vi "Y Axis Motor state control subVI.vi"(8 "error in (no error)":errorcluster, 11 "Y Axis Motor Target":T1) -> (0 "error out":errorcluster, 3 "Y Axis Motor Params":T2)   [LabVIEW 2017]
uses:
  X-Y Manipulator open loop/Control 1.ctl
  Motor Status Enum.ctl
panel:
  in  "Y Axis Motor Target":T1
  in  "stop":bool
  in  "stop 2":bool
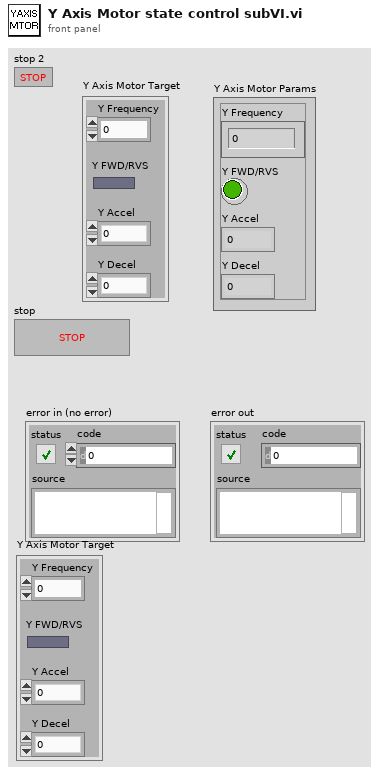
[diagram p1: front panel]
types:
  T1 = typedef "Control 1.ctl" = cluster{"Y Frequency":dbl, "Y FWD/RVS":bool, "Y Accel":dbl, "Y Decel":dbl}
  T2 = cluster{"Y Frequency":dbl, "Y FWD/RVS":bool, "Y Accel":dbl, "Y Decel":dbl}
  T3 = typedef "Motor Status Enum.ctl" = enum16{"Stop Motor", "Read Inputs", "Steady Speed", "Accelerate", "Decelerate"}
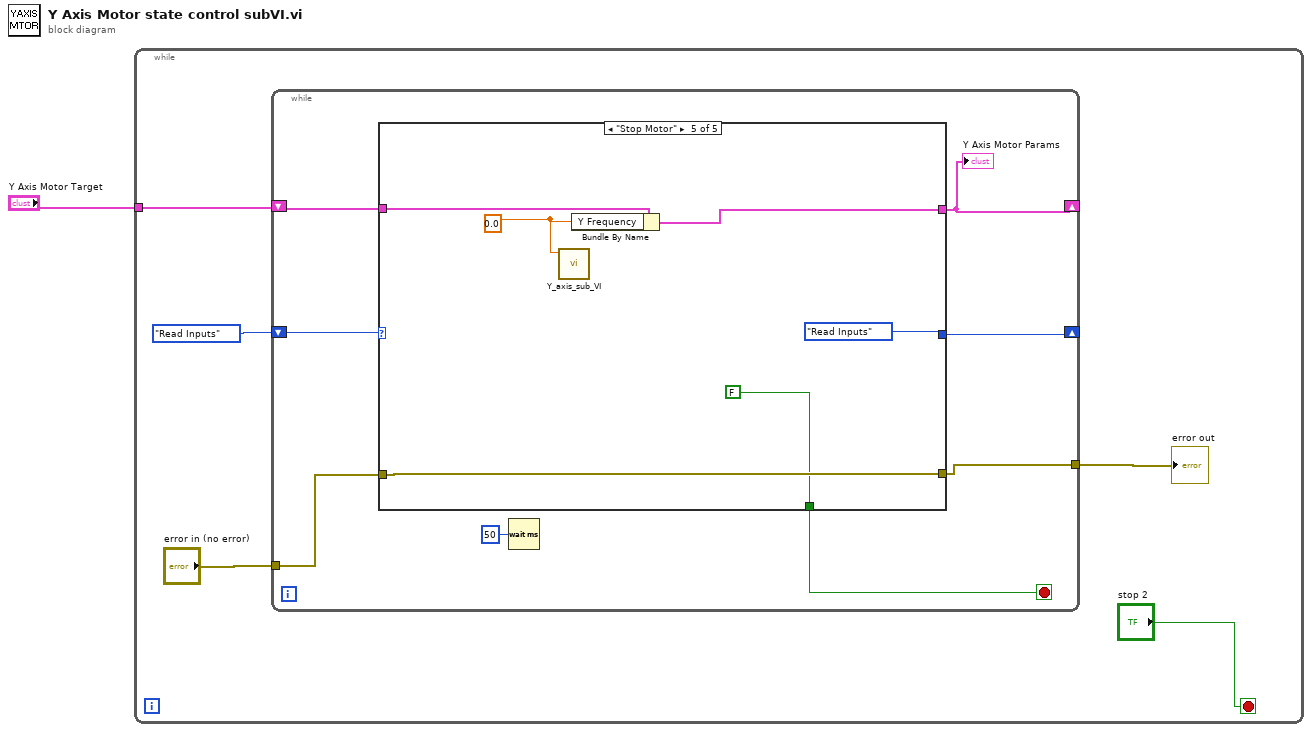
[diagram p0: block diagram]
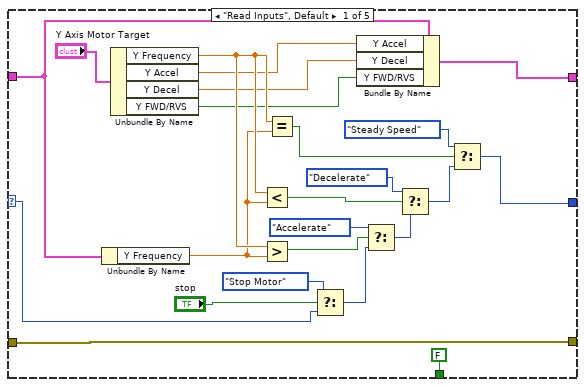
[diagram p2: hidden frame]
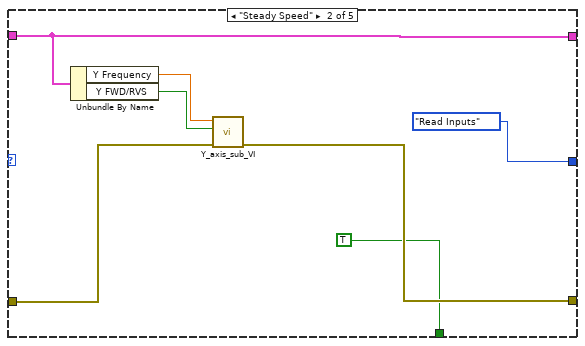
[diagram p3: hidden frame]
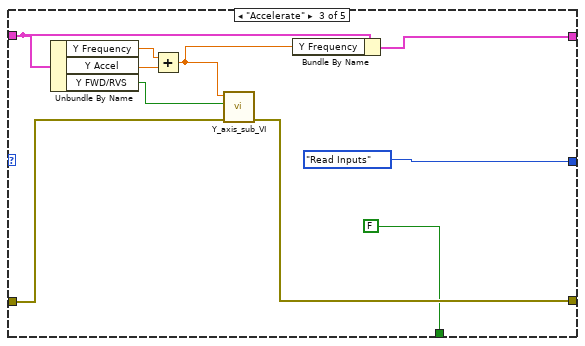
[diagram p4: hidden frame]
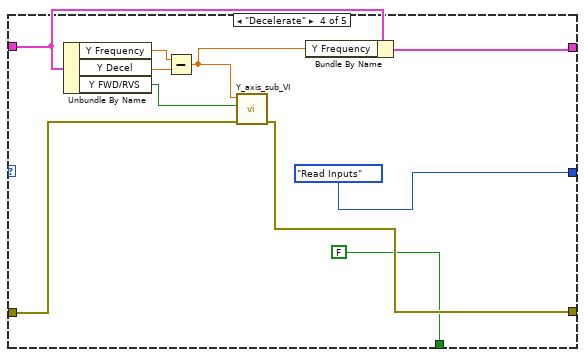
[diagram p5: hidden frame]
diagram:
  n1 = while {
    tunnel: "Y Axis Motor Target" -> [w2]
    stop <- "stop 2" stop-if-true
    n2 = while {
      shift-right: [w14] -> _
      shift-left: Motor_Status_Enum."Read Inputs" -> [w8]
      shift-right: [w12] -> _
      shift-left: w2 -> [w13]
      tunnel: "error in (no error)" -> [w11]
      tunnel: [w10] -> w6
      stop <- w7 stop-if-true
      n3 = case shown="\"Stop Motor\"" w8 {
        selector: w8 -> [w18 _ _ _ _]
        tunnel: [w27 Motor_Status_Enum."Read Inputs" Motor_Status_Enum."Read Inputs" Motor_Status_Enum."Read Inputs" Motor_Status_Enum."Read Inputs"] -> w14
        tunnel: [w25 w40 w50 w61 w70] -> w12
        tunnel: w13 -> [w24 w40 w54 w60 w69]
        tunnel: w11 -> [w26 w44 w52 w59 w67]
        tunnel: [w26 w43 w51 w58 w67] -> w10
        tunnel: [FALSE ("stop") TRUE ("stop") FALSE ("stop") FALSE ("stop") FALSE ("stop")] -> w7
        frame "Read Inputs", Default {
          n4 = Unbundle By Name(w24) -> ("Y Frequency"=w31:dbl)
          n5 = Unbundle By Name("Y Axis Motor Target") -> ("Y Frequency"=w32:dbl, "Y Accel"=w23:dbl, "Y Decel"=w22:dbl, "Y FWD/RVS"=w21:bool)
          n6 = Less?(x=w32, y=w31) -> (x < y?=w35:bool)
          n7 = Greater?(x=w32, y=w31) -> (0:w17:bool)
          n8 = Equal?(x=w32, y=w31) -> (x = y?=w30:bool)
          n9 = Select(t=Motor_Status_Enum."Stop Motor", s="stop", f=w18) -> (s? t:f=w16:T3)
          n10 = Bundle By Name(cluster=w24, "Y Accel"=w23, "Y Decel"=w22, "Y FWD/RVS"=w21) -> (w25:T1)
          n11 = Select(t=Motor_Status_Enum."Accelerate", s=w17, f=w16) -> (s? t:f=w33:T3)
          n12 = Select(t=Motor_Status_Enum."Decelerate", s=w35, f=w33) -> (s? t:f=w29:T3)
          n13 = Select(t=Motor_Status_Enum."Steady Speed", s=w30, f=w29) -> (s? t:f=w27:T3)
        }
        frame "Steady Speed" {
          n14 = Unbundle By Name(w40) -> ("Y Frequency"=w42:dbl, "Y FWD/RVS"=w41:bool)
          n15 = call "Y_axis_sub_VI.vi"("error in (no error)"=w44, "FWD/RVS"=w41, "Frequency"=w42) -> ("error out"=w43:errorcluster)  [unwired: 8 in]
        }
        frame "Accelerate" {
          n16 = Unbundle By Name(w54) -> ("Y Frequency"=w49:dbl, "Y Accel"=w47:dbl, "Y FWD/RVS"=w46:bool)
          n17 = Add(x=w49, y=w47) -> (x+y=w48:dbl)
          n18 = call "Y_axis_sub_VI.vi"("error in (no error)"=w52, "FWD/RVS"=w46, "Frequency"=w48) -> ("error out"=w51:errorcluster)  [unwired: 8 in]
          n19 = Bundle By Name(cluster=w54, "Y Frequency"=w48) -> (w50:T1)
        }
        frame "Decelerate" {
          n20 = Unbundle By Name(w60) -> ("Y Frequency"=w62:dbl, "Y Decel"=w64:dbl, "Y FWD/RVS"=w56:bool)
          n21 = Subtract(x=w62, y=w64) -> (x-y=w63:dbl)
          n22 = call "Y_axis_sub_VI.vi"("error in (no error)"=w59, "FWD/RVS"=w56, "Frequency"=w63) -> ("error out"=w58:errorcluster)  [unwired: 8 in]
          n23 = Bundle By Name(cluster=w60, "Y Frequency"=w63) -> (w61:T1)
        }
        frame "Stop Motor" {
          w68 = 0.0 ("Y Frequency")
          n24 = call "Y_axis_sub_VI.vi"("Frequency"=w68) -> ()  [unwired: 10 in, 1 out]
          n25 = Bundle By Name(cluster=w69, "Y Frequency"=w68) -> (w70:T1)
        }
      }
      "Y Axis Motor Params" <- w12
      n26 = Wait (ms)(milliseconds to wait=u32 50) -> ()  [unwired: 1 out]
    }
    "error out" <- w6
  }
